vi "Project to Plant UML Diagram Script.vi"() -> ()   [LabVIEW 2019]
uses:
  <vilib>/Utility/error.llb/Clear Errors.vi
  <vilib>/Utility/traverseref.llb/Traverse for GObjects.vi
  <vilib>/Utility/Data Type/Get LabVIEW Class Information.vi
panel:
  in  "Classes":i32(listbox)=9
  out "Progress:":dbl(slide)=18.0 caption="Complete" scale=0.0..18.0
  in  "Usage":bool=TRUE
  in  "Composition":bool=TRUE
  in  "Inheritance":bool=TRUE
  out "Plant UML Diagram String":string="Alpha_Task_Msg --|> Message\r\nAlpha_Task_Msg --> Alpha\r\nBeta_Task_Msg --|> Message\r\nBeta_Task_Msg --> Beta\r\nLast_Ack --|> Message\r\nLaunch_Nested_Actor_Msg --|> Message\r\nLog_Event_Msg --|> Message\r\nLog_Event_Msg --> Untitled_Project_1\r\nMessage_Priority_Queue --> Message\r\nMessage_Queue --* Message_Priority_Queue\r\nMessage_Queue --> Message\r\nPing_Msg --|> Message\r\nRegister_Actor_Msg --|> Message\r\nStop_Msg --|> Message\r\nUntitled_Project_1 --> Alpha\r\nUntitled_Project_1 --> Beta\r\n"
  in  "Path":path
  # "http://www.plantuml.com/plantuml/uml"
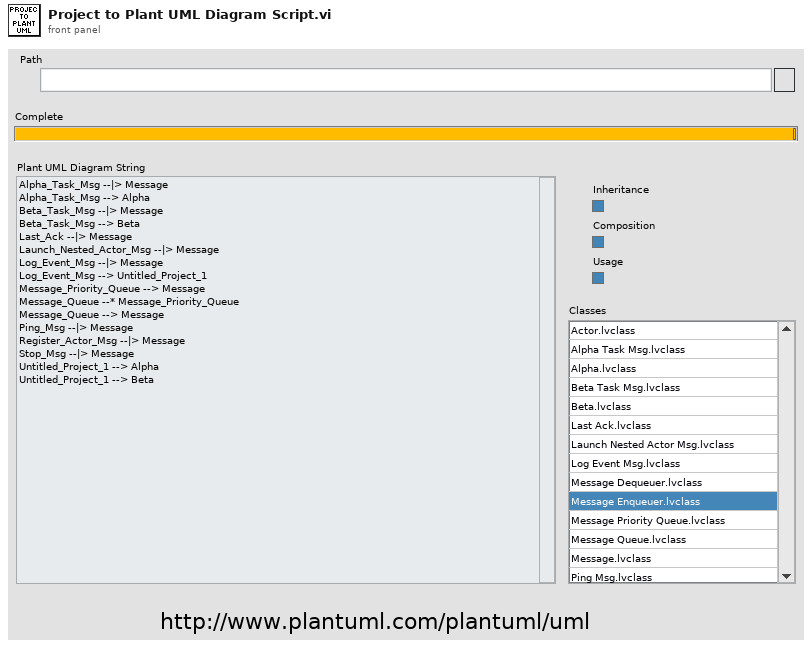
[diagram p1: front panel]
types:
  T1 = map{string, cluster{"Inheritance":set{string}, "Composition":set{string}, "Usage":set{string}}}
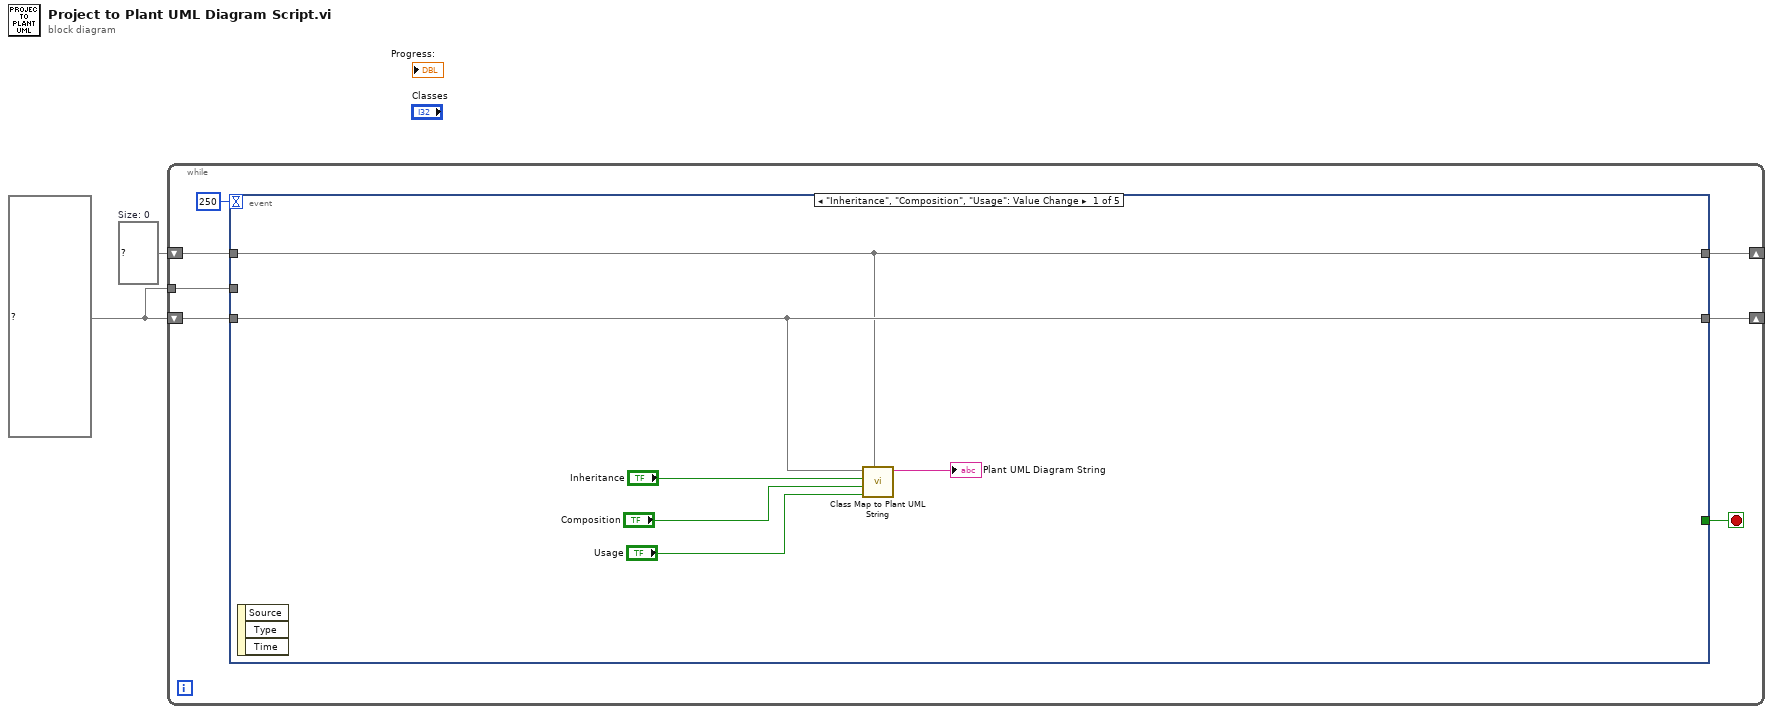
[diagram p0: block diagram]
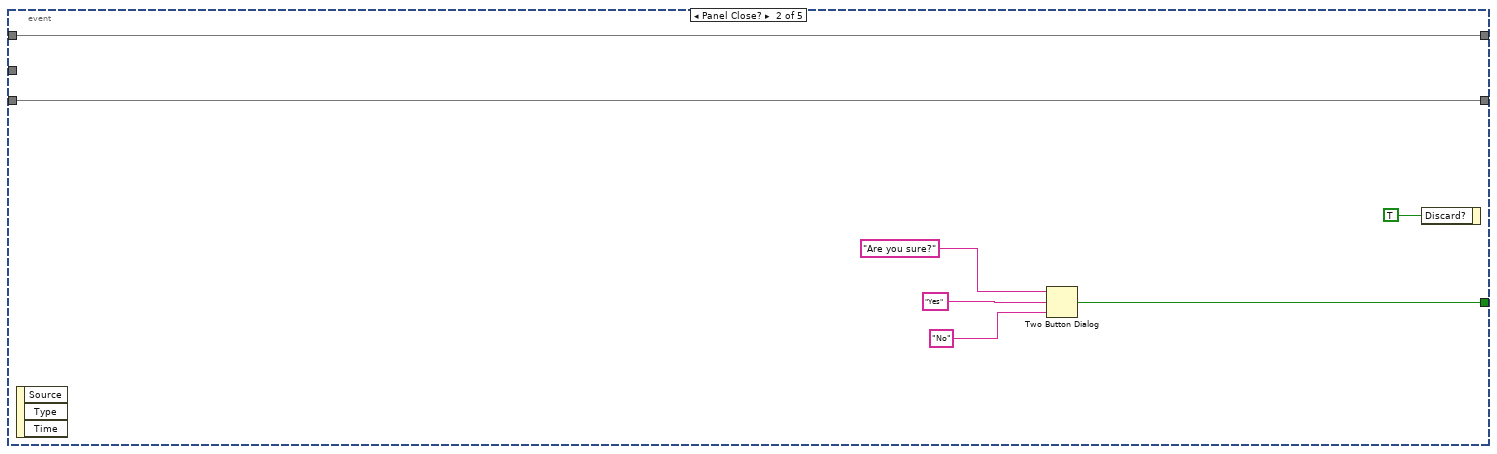
[diagram p2: hidden frame]
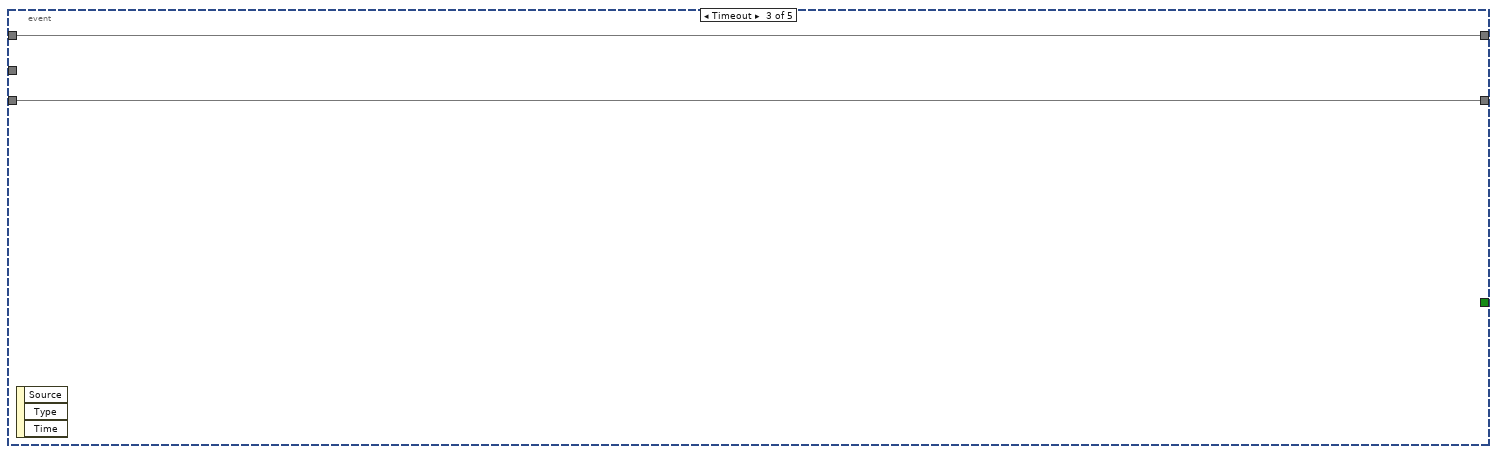
[diagram p3: hidden frame]
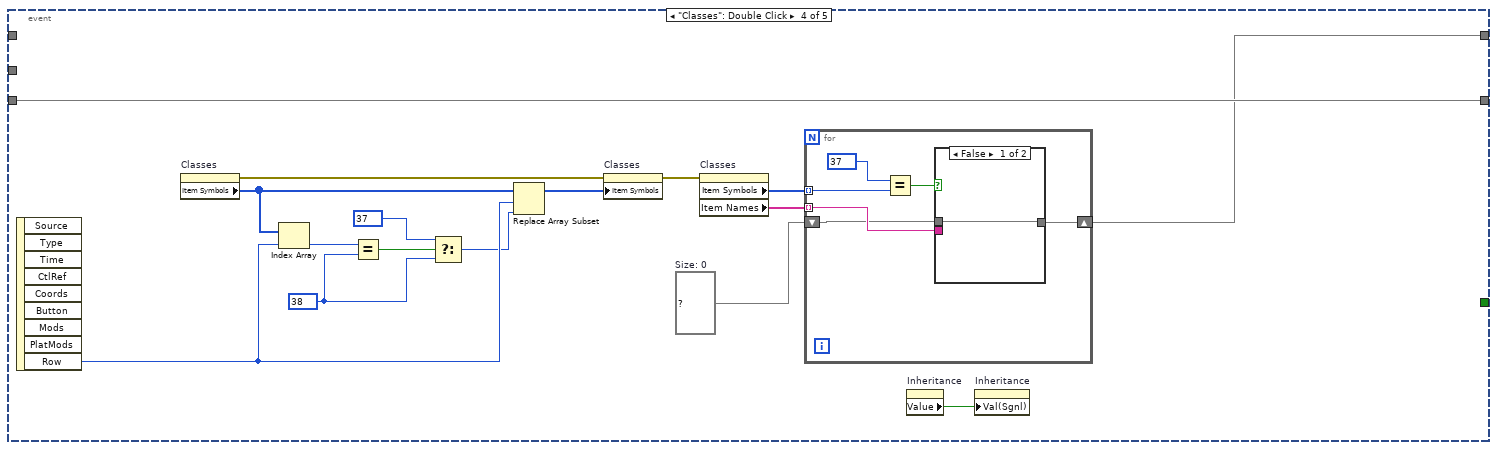
[diagram p4: hidden frame]
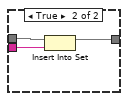
[diagram p5: hidden frame]
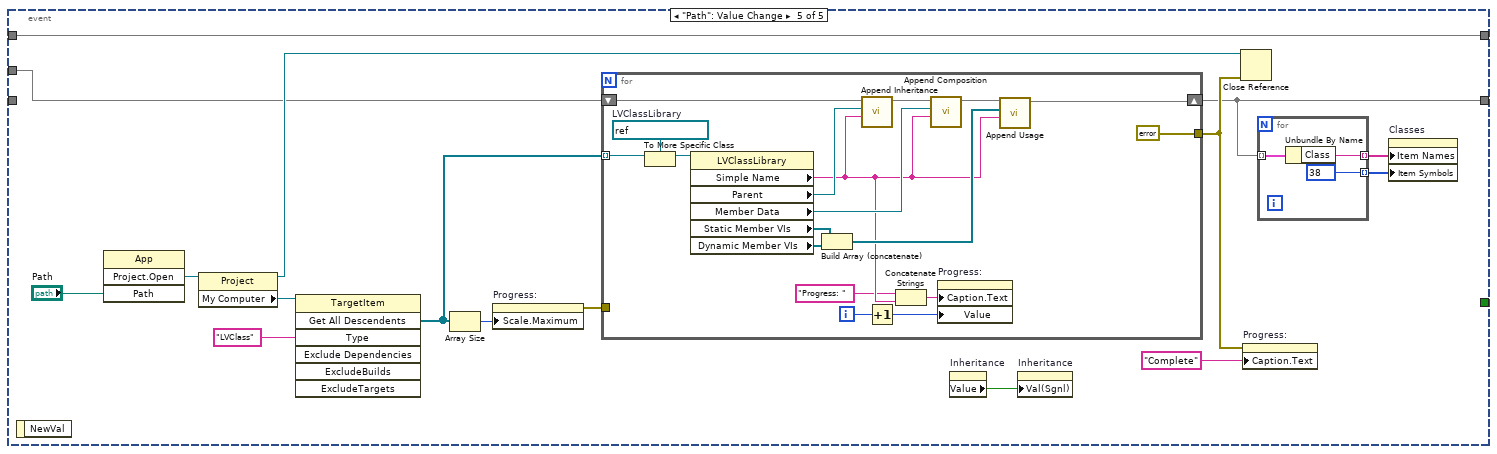
[diagram p6: hidden frame]
diagram:
  w1 = set{string} {}  # Size: 0
  w2 = T1 {} ("map")
  n1 = while {
    shift-right: [w7] -> _
    shift-left: w2 -> [w8]
    tunnel: w2 -> [w6]
    shift-right: [w4] -> _
    shift-left: w1 -> [w3]
    stop <- w5 stop-if-true
    n2 = event shown="[0] \"Inheritance\", \"Composition\", \"Usage\": Value Change" {
      selector: _ -> [_ _ _ _ _]
      dyn-events: _ -> [_ _ _ _ _]
      timeout: 250 -> [_ _ _ _ _]
      tunnel: w8 -> [w11 w21 w24 w35 _]
      tunnel: [w11 w21 w24 w35 w54] -> w7
      tunnel: w6 -> [_ _ _ _ w59]
      tunnel: [_ w17 _ _ _] -> w5
      tunnel: [w10 w16 w23 w26 w52] -> w4
      tunnel: w3 -> [w10 w16 w23 _ w52]
      event "Inheritance", "Composition", "Usage": Value Change {
        n3 = event-data() -> ()  [unwired: 1 in, 3 out]
        n4 = call "Class Map to Plant UML String.vi"("Disabled Set"=w10, "Usage"="Usage", "Composition"="Composition", "Inheritance"="Inheritance", "Class Map"=w11) -> ("Plant UML String"=→"Plant UML Diagram String":string)  [unwired: 6 in]
      }
      event Panel Close? {
        n5 = event-data() -> ()  [unwired: 1 in, 3 out]
        n6 = Two Button Dialog(message="Are you sure?", 1:"No" ("F button name (\"Cancel\")"), 2:"Yes" ("T button name (\"OK\")")) -> (T button?=w17:bool)
        n7 = event-data("Discard?"=TRUE) -> ()  [unwired: 1 in, 1 out]
      }
      event Timeout {
        n8 = event-data() -> ()  [unwired: 1 in, 3 out]
      }
      event "Classes": Double Click {
        w27 = set{string} {}  # Size: 0
        w37 = 38
        n9 = event-data() -> ("Row"=w33:i32)  [unwired: 1 in, 8 out]
        n10 = property on="Classes" class="LstBox (strict)"() -> (error out=w36:errorcluster, "Item Symbols"=w34:i32[])  [unwired: 2 in, 1 out]
        n11 = Index Array(array=w34, index=w33) -> (element=w40:i32)
        n12 = Equal?(x=w40, y=w37) -> (x = y?=w39:bool)
        n13 = Select(t=37, s=w39, f=w37) -> (s? t:f=w32:i32)
        n14 = Replace Array Subset(array=w34, new element=w32, index=w33) -> (w31:i32[])
        n15 = property on="Classes" class="LstBox (strict)"(error in=w36, "Item Symbols"=w31) -> (error out=w30:errorcluster)  [unwired: 1 in, 1 out]
        n16 = property on="Classes" class="LstBox (strict)"(error in=w30) -> ("Item Symbols"=w29:i32[], "Item Names"=w28:string[])  [unwired: 1 in, 2 out]
        n17 = for {
          tunnel: w29 -> [w46] mode=indexing
          tunnel: w28 -> [w43] mode=indexing
          shift-right: [w42] -> w26
          shift-left: w27 -> [w41]
          n18 = Equal?(x=37, y=w46) -> (x = y?=w44:bool)
          n19 = case shown="False" w44 {
            tunnel: w43 -> [_ w50]
            tunnel: [w47 w49] -> w42
            tunnel: w41 -> [w47 w48]
            frame False {
            }
            frame True {
              n20 = Insert Into Set(10:w50, 11:w48) -> (3:w49:set{string})  [unwired: 1 out]
            }
          }
        }
        n21 = property on="Inheritance" class="Bool (strict)"() -> ("Value"=w25:bool)  [unwired: 2 in, 2 out]
        n22 = property on="Inheritance" class="Bool (strict)"("Val(Sgnl)"=w25) -> ()  [unwired: 2 in, 2 out]
      }
      event "Path": Value Change {
        n23 = event-data() -> ()  [unwired: 1 in, 1 out]
        n24 = invoke class="App" method="Project.Open"("Path"="Path") -> ("Project:Open"=w65:refnum<vi>)  [unwired: 3 in, 3 out]
        n25 = property class="Project"(reference=w65) -> (reference out=w60:refnum<vi>, "My Computer"=w66:refnum<vi>)  [unwired: 1 in, 1 out]
        n26 = invoke class="TargetItem" method="Get All Descendents"(reference=w66, "Type"="LVClass") -> ("All Descendents"=w61:refnum<vi>[])  [unwired: 5 in, 6 out]
        n27 = Array Size(array=w61) -> (size(s)=w57:i32)
        n28 = property on="Progress:" class="Slide (strict)"("Scale.Maximum"=w57) -> (error out=w62:errorcluster)  [unwired: 2 in, 1 out]
        n29 = for {
          tunnel: w61 -> [w87] mode=indexing
          shift-right: [w77] -> w54
          shift-left: w59 -> [w80]
          tunnel: [errorcluster {"status"=FALSE, "code"=0, "source"=""} ("error constant")] -> w56
          tunnel: w62 -> [_]
          i -> [w73]
          w86 = refnum<vi> refnum  # LVClassLibrary
          n30 = To More Specific Class(target class=w86, reference=w87) -> (specific class reference=w85:refnum<vi>)  [unwired: 1 in, 1 out]
          n31 = property class="LVClassLibrary"(reference=w85) -> ("Simple Name"=w75:string, "Parent"=w79:refnum<vi>, "Member Data"=w81:refnum<vi>, "Static Member VIs"=w84:refnum<vi>[], "Dynamic Member VIs"=w83:refnum<vi>[])  [unwired: 1 in, 2 out]
          n32 = Build Array (concatenate)(w84, w83) -> (w82:refnum<vi>[])
          n33 = call "Append Inheritance.vi"("Class"=w75, "Parent Class"=w79, "Class Relations Map"=w80) -> ("Class Relations Map Out"=w71:T1)  [unwired: 8 in]
          n34 = Increment(x=w73) -> (x+1=w70:i32)
          n35 = Concatenate Strings("Progress: " ("string"), w75) -> (w76:string)
          n36 = call "Append Composition.vi"("Class"=w75, "Private Data Control"=w81, "Class Relations Map"=w71) -> ("Class Relations Map Out"=w72:T1)  [unwired: 8 in]
          n37 = property on="Progress:" class="Slide (strict)"("Caption.Text"=w76, "Value"=w70) -> ()  [unwired: 2 in, 2 out]
          n38 = call "Append Usage.vi"("Class"=w75, "VIs"=w82, "Class Relations Map"=w72) -> ("Class Relations Map Out"=w77:T1)  [unwired: 8 in]
        }
        n39 = property on="Inheritance" class="Bool (strict)"() -> ("Value"=w51:bool)  [unwired: 2 in, 2 out]
        n40 = property on="Inheritance" class="Bool (strict)"("Val(Sgnl)"=w51) -> ()  [unwired: 2 in, 2 out]
        n41 = Close Reference(reference=w60, error in (no error)=w56) -> ()  [unwired: 1 out]
        n42 = property on="Progress:" class="Slide (strict)"(error in=w56, "Caption.Text"="Complete") -> ()  [unwired: 1 in, 2 out]
        n43 = for {
          tunnel: [w68] -> w55 mode=indexing
          tunnel: w54 -> [w69] mode=indexing
          tunnel: [38] -> w53 mode=indexing
          n44 = Unbundle By Name(w69) -> ("Class"=w68:string)
        }
        n45 = property on="Classes" class="LstBox (strict)"("Item Names"=w55, "Item Symbols"=w53) -> ()  [unwired: 2 in, 2 out]
      }
    }
  }
